vi "Write Extinction.vi"(8 "error in (no error)":errorcluster, 10 "Extinction":cluster{"Mean":dbl, "Error":dbl}[](array[cluster]), 11 "State Data in":refnum<class "State Data.lvclass">) -> (0 "error out":errorcluster, 3 "State Data out":refnum<class "State Data.lvclass">)   [LabVIEW 2015, in "State Data.lvclass"]
uses:
  State Data.lvclass
  State Data.lvclass/State Data.ctl
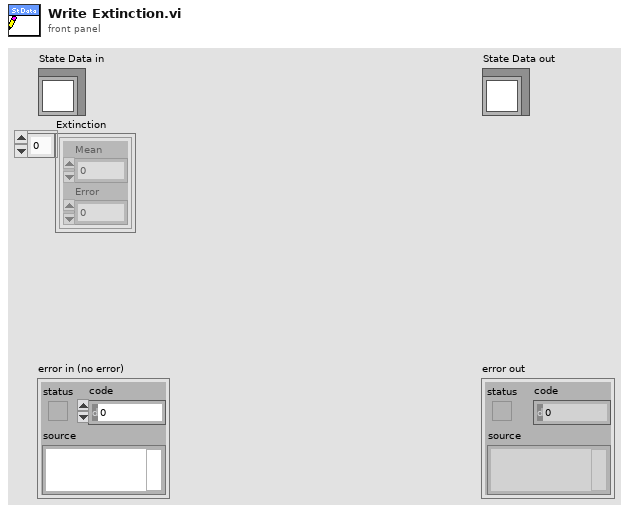
[diagram p1: front panel]
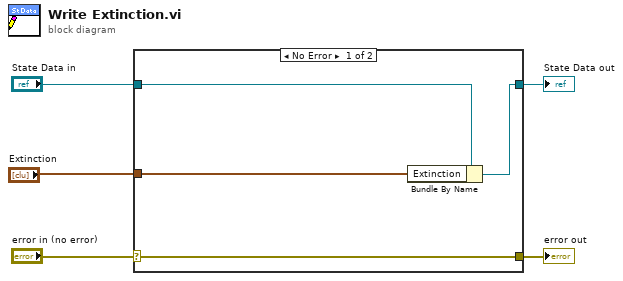
[diagram p0: block diagram]
diagram:
  n1 = case shown="No Error" "error in (no error)" {
    selector: "error in (no error)" -> [w9 w10]
    tunnel: [w9 w10] -> w4
    tunnel: [w7 w11] -> w2
    tunnel: "State Data in" -> [w8 w11]
    tunnel: "Extinction" -> [w6 _]
    frame No Error {
      n2 = Bundle By Name(cluster=w8, "Extinction"=w6) -> (w7:refnum<class "State Data.lvclass">)
    }
    frame Error {
    }
  }
  "error out" <- w4
  "State Data out" <- w2
